vi "APC_9056_MaskErrors.vi"(1 "UnMaskedWarning":u8[](array[numeric]), 2 "rastermask":bool[](array[boolean])) -> (0 "MaskedWarning":u8[](array[numeric]))   [LabVIEW 2020]
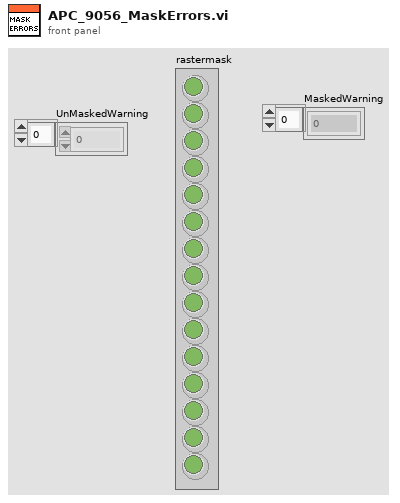
[diagram p1: front panel]
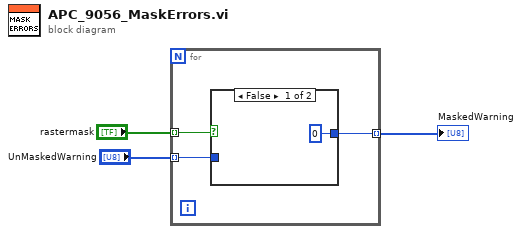
[diagram p0: block diagram]
diagram:
  n1 = for {
    tunnel: [w6] -> w3 mode=indexing
    tunnel: "UnMaskedWarning" -> [w5] mode=indexing
    tunnel: "rastermask" -> [w4] mode=indexing
    n2 = case shown="False" w4 {
      tunnel: [u8 0 ("Numeric") w8] -> w6
      tunnel: w5 -> [_ w8]
      frame False {
      }
      frame True {
      }
    }
  }
  "MaskedWarning" <- w3
